vi "ITR_6008.vi"() -> ()   [LabVIEW 2020]
uses:
  <vilib>/Instr/_visa.llb/VISA Configure Serial Port (Instr).vi
panel:
  out "Numeric":dbl
  in  "stop":bool
  in  "VISA resource name":refnum<visa-resource-name>
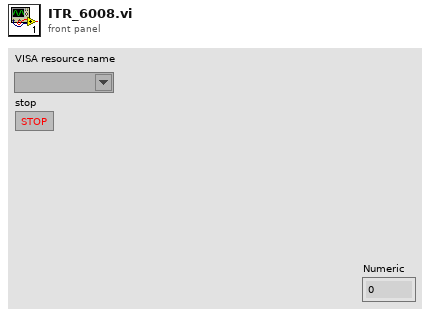
[diagram p1: front panel]
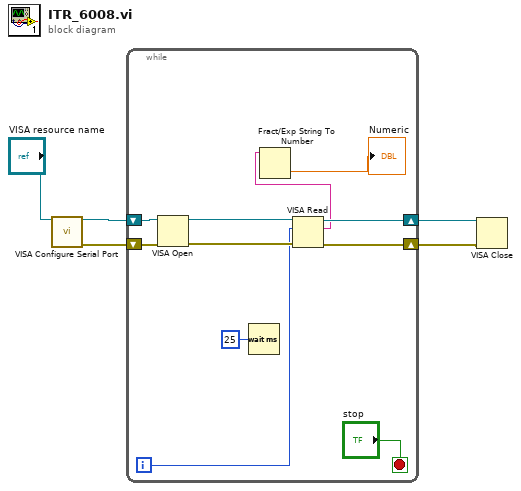
[diagram p0: block diagram]
diagram:
  n1 = call-poly "VISA Configure Serial Port"("VISA resource name"="VISA resource name") -> ("VISA resource name out"=w5:refnum<visa-resource-name>, "error out"=w3:errorcluster)  [unwired: 13 in]
  n2 = while {
    shift-right: [w14] -> w4
    shift-left: w5 -> [w16]
    shift-right: [w11] -> w2
    shift-left: w3 -> [w13]
    i -> [w6]
    stop <- "stop" stop-if-true
    n3 = VISA Open(error in (no error)=w13, VISA resource name=w16) -> (VISA resource name=w15:refnum<visa-resource-name>, error out=w12:errorcluster)  [unwired: 3 in]
    n4 = Wait (ms)(milliseconds to wait=u32 25) -> ()  [unwired: 1 out]
    n5 = VISA Read(VISA resource name=w15, byte count=w6, error in (no error)=w12) -> (VISA resource name out=w14:refnum<visa-resource-name>, read buffer=w9:string, error out=w11:errorcluster)  [unwired: 1 out]
    n6 = Fract/Exp String To Number(string=w9) -> (number=→"Numeric":dbl)  [unwired: 3 in, 1 out]
  }
  n7 = VISA Close(VISA resource name=w4, error in (no error)=w2) -> ()  [unwired: 1 out]
